vi "Image_get.vi"(8 "error in (no error)":errorcluster) -> (0 "error out":errorcluster, 2 "Image":T1)   [LabVIEW 2009, in "NetworkVarTarget.lvlib"]
uses:
  NetworkVarTarget.lvlib
  <vilib>/vision/Image Controls.llb/IMAQ Image.ctl
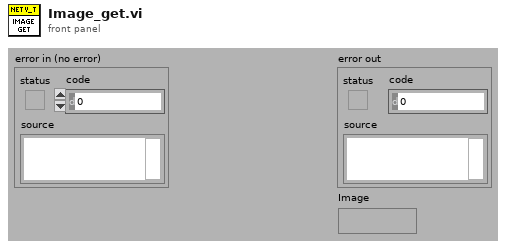
[diagram p1: front panel]
types:
  T1 = typedef "IMAQ Image.ctl" = refnum<image>
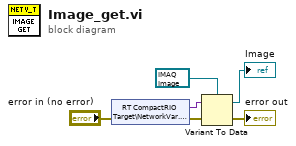
[diagram p0: block diagram]
diagram:
  n1 = shared-variable "RT CompactRIO Target\\NetworkVar.lvlib\\Image"(error in="error in (no error)") -> (w4:variant, error out=w2:errorcluster)
  n2 = Variant To Data(error in=w2, Variant=w4, type=T1 refnum ("Image 2")) -> (error out=→"error out":errorcluster, data=→"Image":T1)
